vi "Wii_3D_mapping.vi"(0 "Wii_X_off":dbl, 1 "previous_X_3D":dbl, 2 "previous_Y_3D":dbl, 3 "previous_Z_3D":dbl, 5 "Wii_Y_off":dbl, 9 "Wii_Z_off":dbl, 12 "X_Y_speed":dbl, 13 "Z_speed":dbl) -> (4 "X_3D":dbl, 6 "Y_3D":dbl, 10 "Z_3D":dbl)   [LabVIEW 2011]
panel:
  out "Zmax":dbl=2.5
  out "X_resolution":i16
  out "Y_resolution":i16
  out "Ymax":dbl
  out "Xmax":dbl=2.5
  out "Y_scaling":dbl
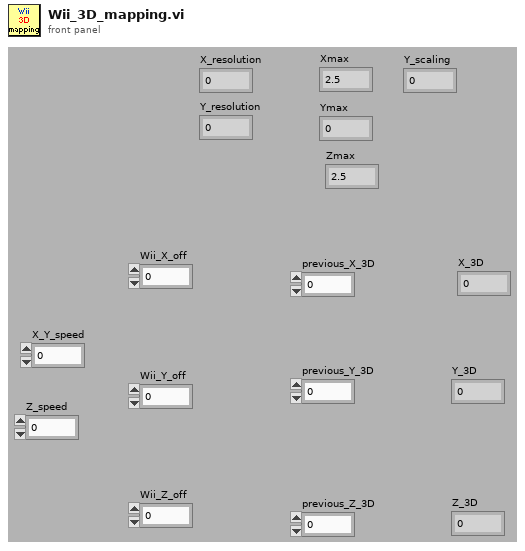
[diagram p1: front panel]
types:
  T1 = typedef "LVAllMonitorsDisplayTypeDef.ctl" = cluster{"Bounds":cluster{"Left":i16, "Top":i16, "Right":i16, "Bottom":i16}, "Depth":i16}[]
  T2 = cluster{"Bounds":cluster{"Left":i16, "Top":i16, "Right":i16, "Bottom":i16}, "Depth":i16}
  T3 = cluster{"Left":i16, "Top":i16, "Right":i16, "Bottom":i16}
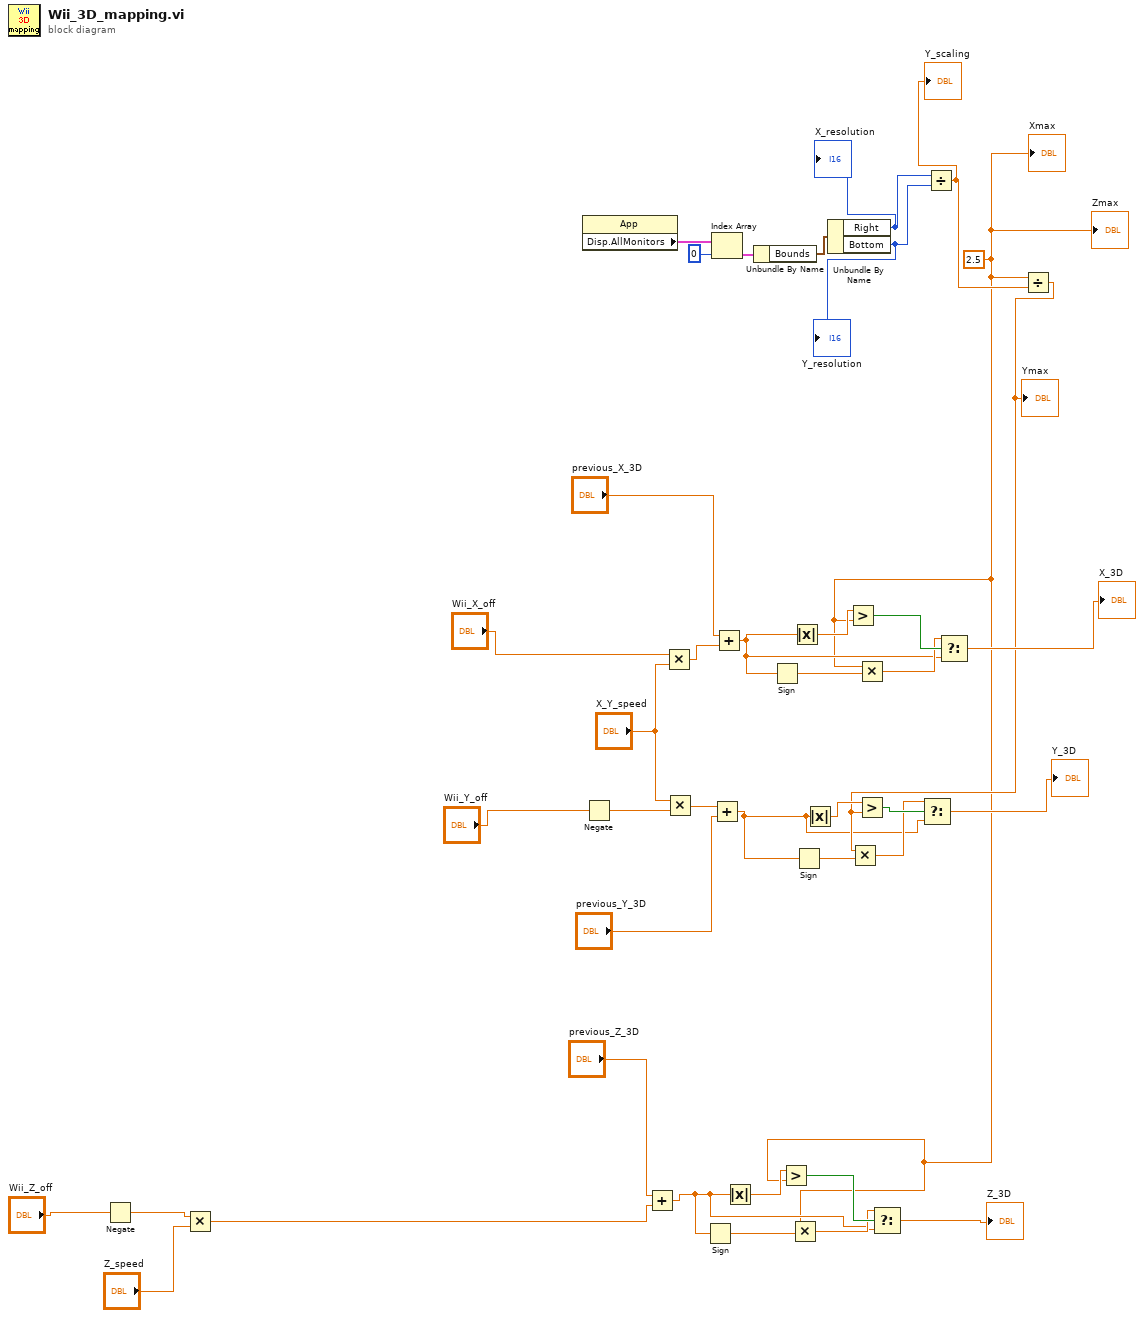
[diagram p0: block diagram]
diagram:
  w4 = 2.5 ("x")
  n1 = Negate(x="Wii_Z_off") -> (-x=w2:dbl)
  n2 = Multiply(x=w2, y="Z_speed") -> (x*y=w1:dbl)
  n3 = property class="App"() -> ("Disp.AllMonitors"=w38:T1)  [unwired: 2 in, 2 out]
  n4 = Negate(x="Wii_Y_off") -> (-x=w3:dbl)
  n5 = Add(x="previous_Z_3D", y=w1) -> (x+y=w11:dbl)
  n6 = Multiply(x="Wii_X_off", y="X_Y_speed") -> (x*y=w33:dbl)
  n7 = Multiply(x="X_Y_speed", y=w3) -> (x*y=w31:dbl)
  n8 = Sign(1:w11) -> (0:w13:dbl)
  n9 = Index Array(array=w38, index=u16 0 ("Front Panel Window:Monitor")) -> (element=w40:T2)
  n10 = Add(x=w31, y="previous_Y_3D") -> (x+y=w18:dbl)
  n11 = Add(x="previous_X_3D", y=w33) -> (x+y=w24:dbl)
  n12 = Absolute Value(x=w11) -> (abs(x)=w15:dbl)
  n13 = Unbundle By Name(w40) -> ("Bounds"=w37:T3)
  n14 = Sign(1:w24) -> (0:w27:dbl)
  n15 = Greater?(x=w15, y=w4) -> (0:w14:bool)
  n16 = Multiply(x=w4, y=w13) -> (x*y=w12:dbl)
  n17 = Absolute Value(x=w24) -> (abs(x)=w29:dbl)
  n18 = Sign(1:w18) -> (0:w20:dbl)
  n19 = Absolute Value(x=w18) -> (abs(x)=w23:dbl)
  n20 = Unbundle By Name(w37) -> ("Right"=w35:i16, "Bottom"=w36:i16)
  "Y_resolution" <- w36
  "X_resolution" <- w35
  n21 = Greater?(x=w29, y=w4) -> (0:w28:bool)
  n22 = Multiply(x=w4, y=w27) -> (x*y=w26:dbl)
  n23 = Select(t=w12, s=w14, f=w11) -> (s? t:f=→"Z_3D":dbl)
  n24 = Divide(x=w35, y=w36) -> (x/y=w34:dbl)
  "Y_scaling" <- w34
  n25 = Select(t=w26, s=w28, f=w24) -> (s? t:f=→"X_3D":dbl)
  n26 = Divide(x=w4, y=w34) -> (x/y=w21:dbl)
  "Ymax" <- w21
  n27 = Multiply(x=w21, y=w20) -> (x*y=w19:dbl)
  n28 = Greater?(x=w23, y=w21) -> (0:w22:bool)
  n29 = Select(t=w19, s=w22, f=w18) -> (s? t:f=→"Y_3D":dbl)
  "Xmax" <- w4
  "Zmax" <- w4
